vi "temp_probe_set_initialize.vi"(6 "Thermal Coefficient Path":path, 8 "error in (no error)":errorcluster, 11 "TempProbeSet in":refnum<class "TempProbeSet.lvclass">) -> (0 "error out":errorcluster, 3 "TempProbeSet out":refnum<class "TempProbeSet.lvclass">)   [LabVIEW 2010, in "TempProbeSet.lvclass"]
uses:
  TempProbeSet.lvclass
  TempProbe.lvclass
  <vilib>/Utility/file.llb/Read From Spreadsheet File (string).vi
panel:
  out "Thermal Coeffient Array":string[][](array[string])
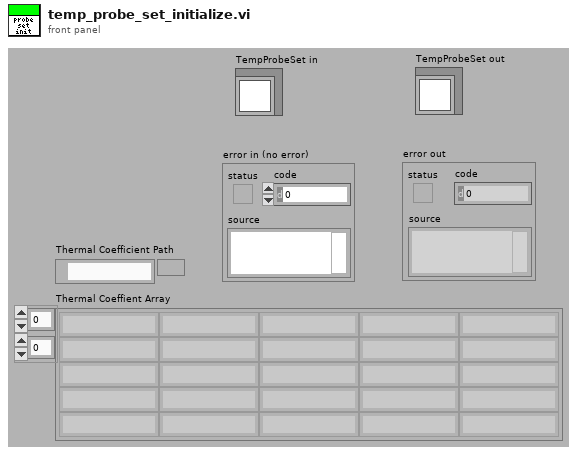
[diagram p1: front panel]
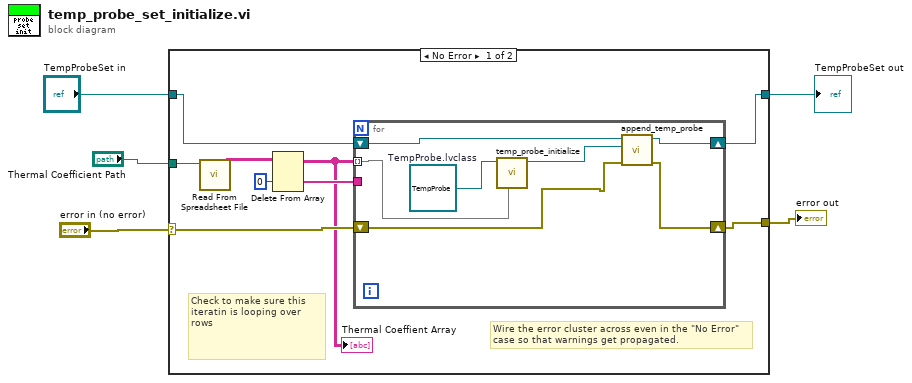
[diagram p0: block diagram]
diagram:
  n1 = case shown="No Error" "error in (no error)" {
    selector: "error in (no error)" -> [w8 w23]
    tunnel: [w9 w23] -> w4
    tunnel: [w10 w22] -> w1
    tunnel: "TempProbeSet in" -> [w6 w22]
    tunnel: "Thermal Coefficient Path" -> [w14 _]
    frame No Error {
      # "Check to make sure this iteratin is looping over rows"
      # "Wire the error cluster across even in the \"No Error\"\ncase so that warnings get propagated."
      n2 = call-poly <vilib>:"Read From Spreadsheet File.vi"("file path (dialog if empty)"=w14) -> ("all rows"=w13:string[][])  [unwired: 6 in, 4 out]
      n3 = Delete From Array(array=w13, index (row)=0) -> (deleted portion=w11:string[], array with subset deleted=w7:string[][])  [unwired: 2 in]
      "Thermal Coeffient Array" <- w7
      n4 = for {
        tunnel: w7 -> [w20] mode=indexing
        tunnel: w11 -> [_]
        shift-right: [w18] -> w9
        shift-left: w8 -> [w16]
        shift-right: [w19] -> w10
        shift-left: w6 -> [w15]
        w21 = refnum<class "TempProbe.lvclass"> refnum  # TempProbe.lvclass
        n5 = call "temp_probe_initialize.vi"("probe data"=w20, "TempProbe in"=w21) -> ("TempProbe out"=w17:refnum<class "TempProbe.lvclass">)  [unwired: 8 in, 1 out]
        n6 = call "append_temp_probe.vi"("error in (no error)"=w16, "TempProbe in"=w17, "TempProbeSet in"=w15) -> ("error out"=w18:errorcluster, "TempProbeSet out"=w19:refnum<class "TempProbeSet.lvclass">)  [unwired: 7 in]
      }
    }
    frame Error {
    }
  }
  "error out" <- w4
  "TempProbeSet out" <- w1
